vi "Read VehicleID.vi"(8 "error in (no error)":errorcluster, 11 "Vehicle in":refnum<class "Vehicle.lvclass">) -> (0 "error out":errorcluster, 2 "VehicleID":i32, 3 "Vehicle out":refnum<class "Vehicle.lvclass">)   [LabVIEW 2020, in "ORM_Examples.lvlib" / "Vehicle.lvclass"]
uses:
  Vehicle.lvclass
  Vehicle.lvclass/Vehicle.ctl
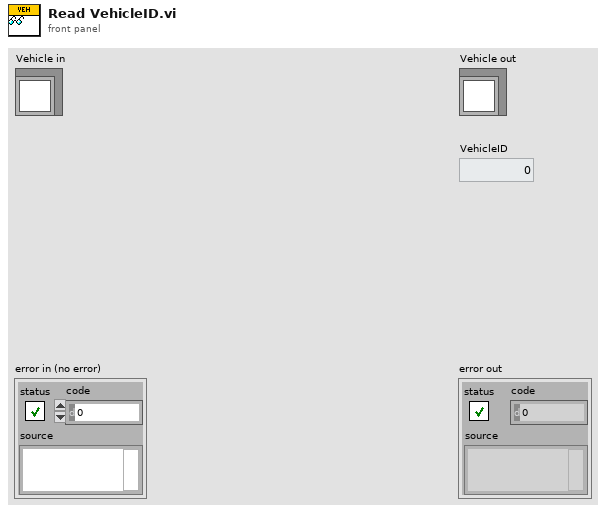
[diagram p1: front panel]
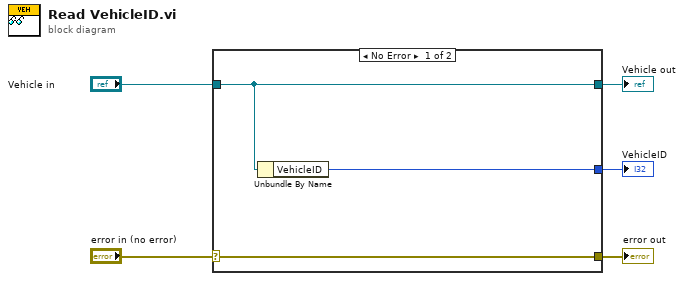
[diagram p0: block diagram]
diagram:
  n1 = case shown="No Error" "error in (no error)" {
    selector: "error in (no error)" -> [w8 w9]
    tunnel: [w8 w9] -> w4
    tunnel: [w7 w10] -> w2
    tunnel: "Vehicle in" -> [w7 w10]
    tunnel: [w6 _] -> w1
    frame No Error {
      n2 = Unbundle By Name(w7) -> ("VehicleID"=w6:i32)
    }
    frame Error {
    }
  }
  "error out" <- w4
  "Vehicle out" <- w2
  "VehicleID" <- w1
